vi "graph_2d.vi"() -> ()   [LabVIEW 2020]
uses:
  <vilib>/Analysis/1siggen.llb/Ramp Pattern by Samples.vi
  <vilib>/Analysis/NI_AALBase.lvlib
panel:
  out "graph":dbl[][](graph)
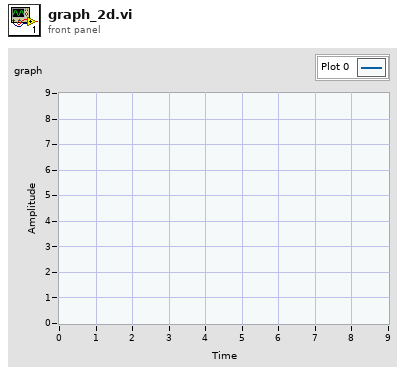
[diagram p1: front panel]
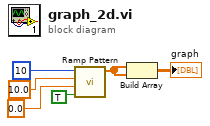
[diagram p0: block diagram]
diagram:
  n1 = call-poly <vilib>:"Ramp Pattern.vi"("exclude end?"=TRUE, "start"=0.0, "end"=10.0, "samples"=10) -> ("Ramp Pattern"=w2:dbl[])  [unwired: 6 in, 1 out]
  n2 = Build Array(w2, w2) -> (→"graph":dbl[][])
